vi "CC Hardware Config Dialog.vi"() -> (3 "Hardware Config":T1)   [LabVIEW 2024]
uses:
  typedefs/CC cluster Hardware Config.ctl
  typedefs/CC cluster Device Index.ctl
panel:
  in  "Edit":bool
  in  "Remove Type":bool
  in  "Add New Type":bool
  in  "Update":bool
  in  "Types":u16(ring) items=["Simulation", "RIMAS"]
  in  "Installed Hardware":i32(listbox)
  in  "Cancel Button":bool
  in  "OK Button":bool
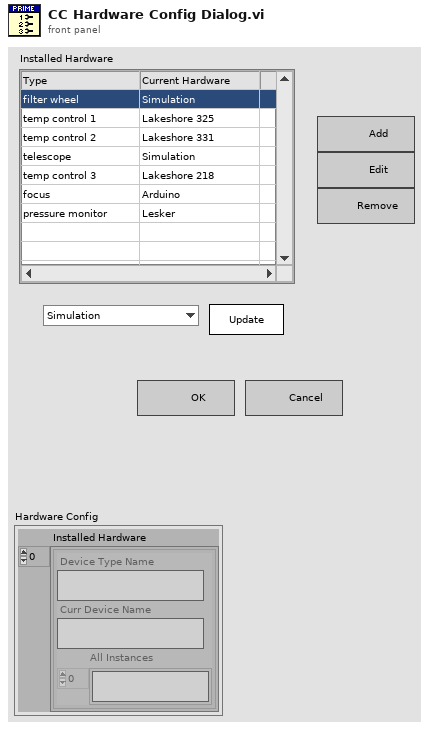
[diagram p1: front panel]
types:
  T1 = typedef "CC cluster Hardware Config.ctl" = cluster{"Installed Hardware":T2[]}
  T2 = typedef "CC cluster Device Index.ctl" = cluster{"Device Type Name":string, "Curr Device Name":string, "All Instances":string[]}
  T3 = cluster{"state":refnum<user-event>, "Hardware Config":T1}
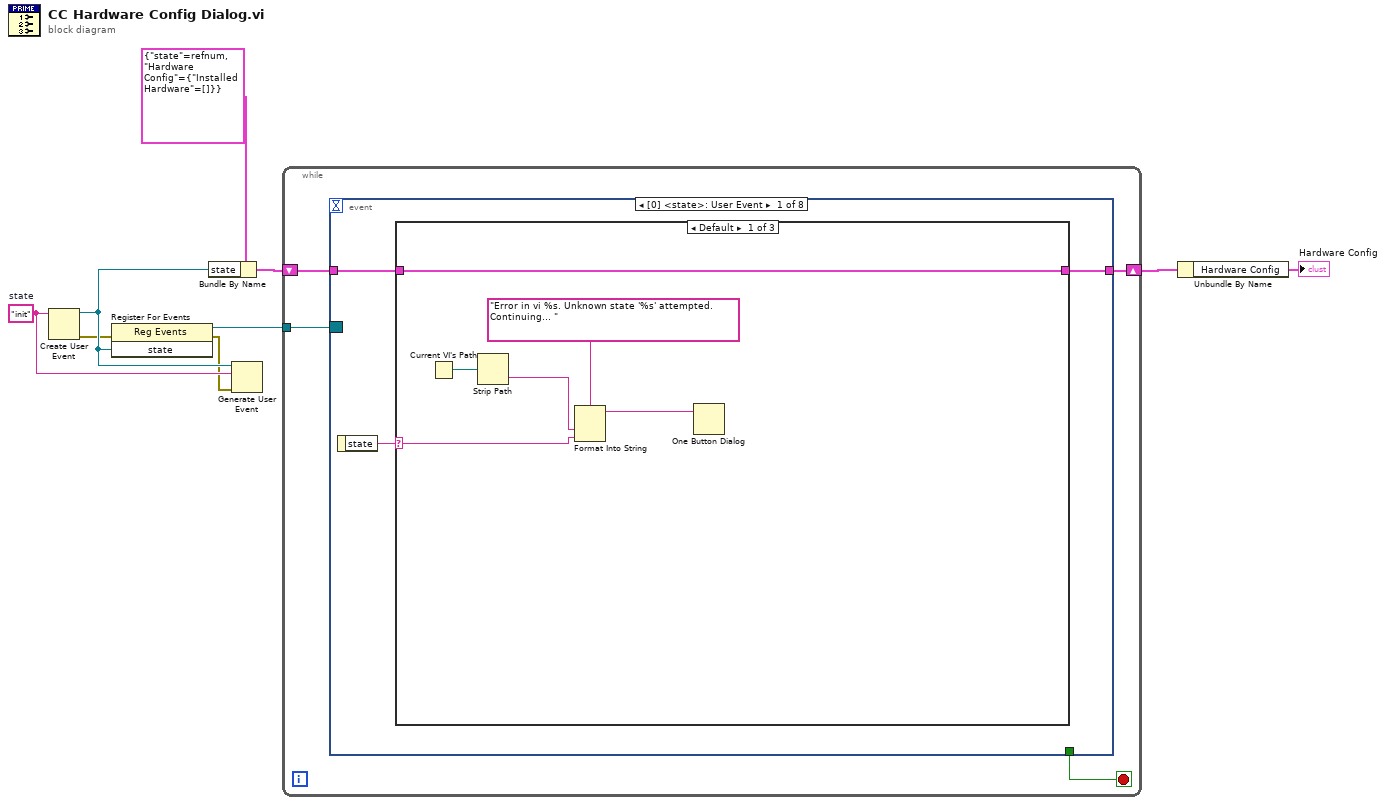
[diagram p0: block diagram]
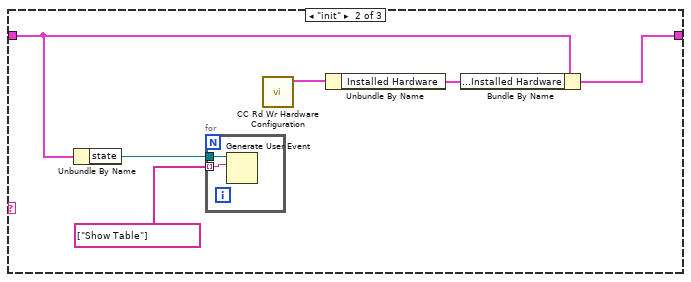
[diagram p2: hidden frame]
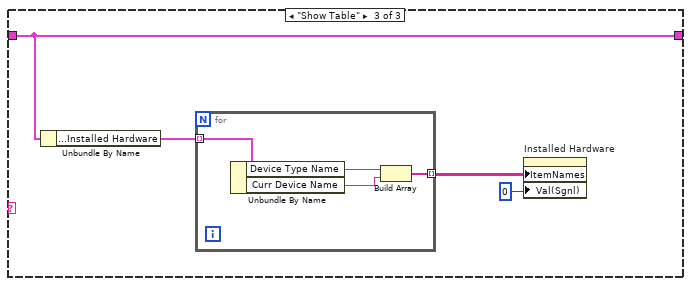
[diagram p3: hidden frame]
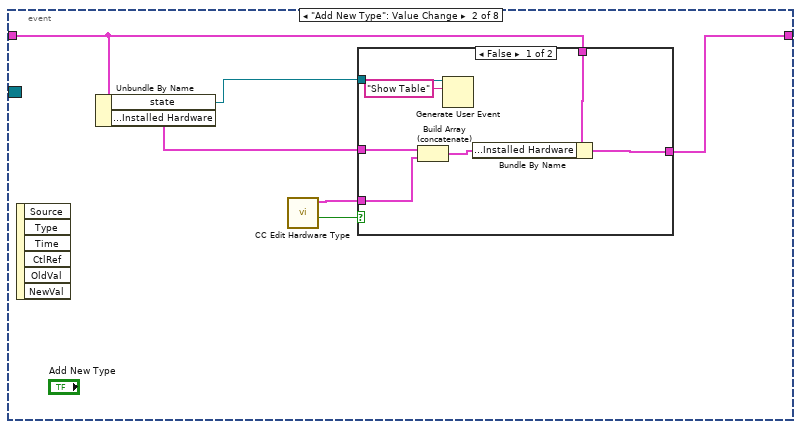
[diagram p4: hidden frame]
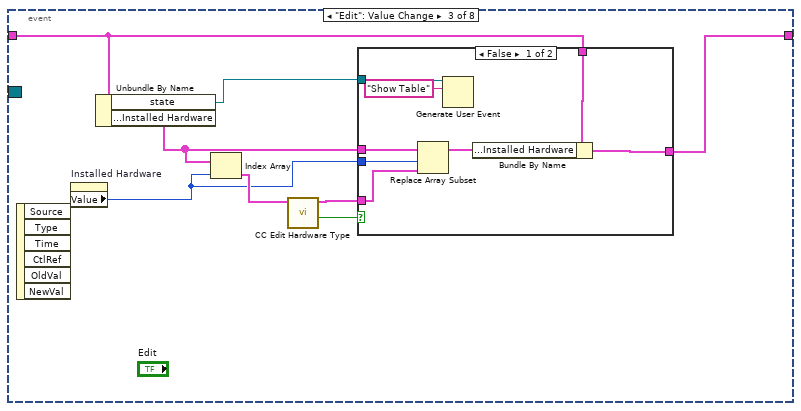
[diagram p6: hidden frame]
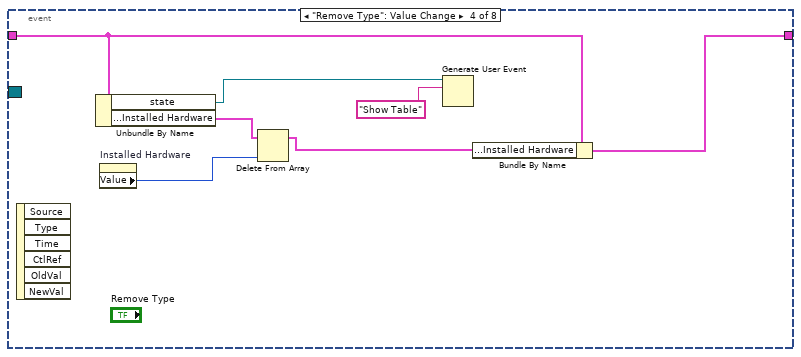
[diagram p8: hidden frame]
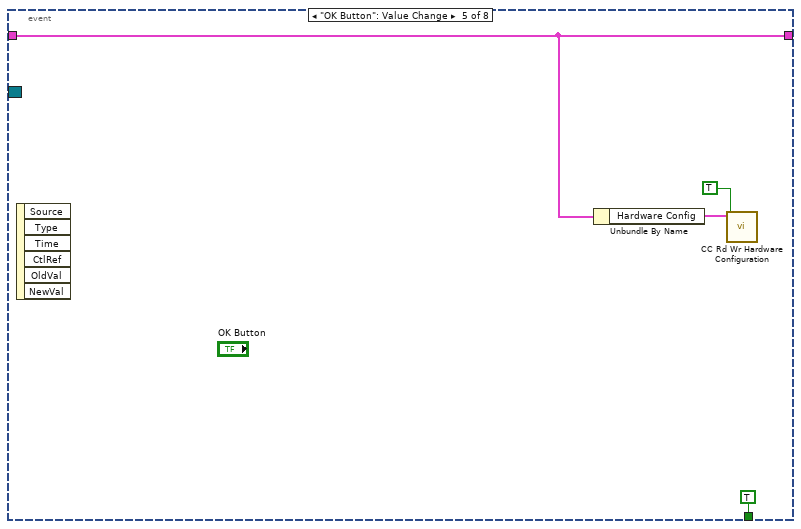
[diagram p9: hidden frame]
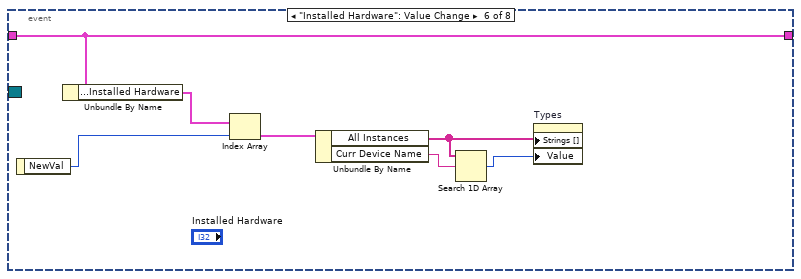
[diagram p10: hidden frame]
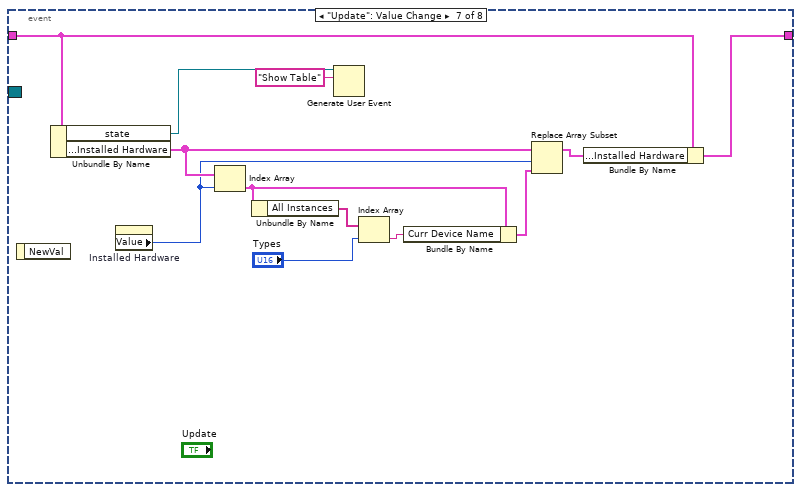
[diagram p11: hidden frame]
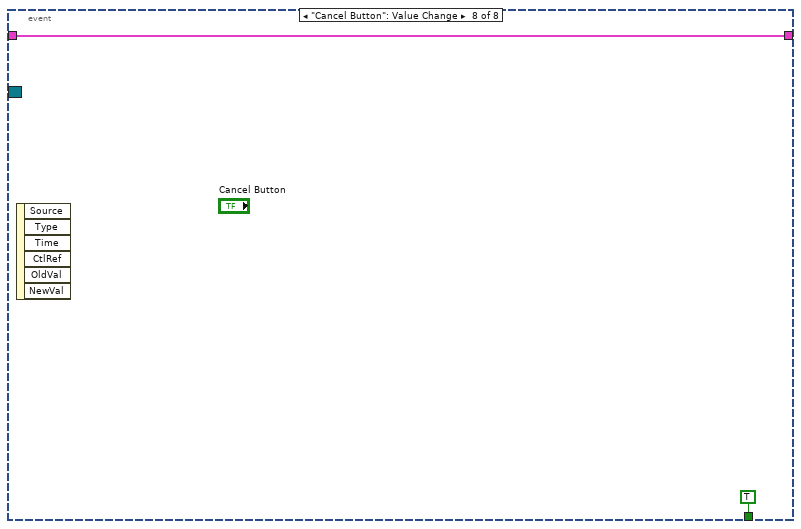
[diagram p12: hidden frame]
diagram:
  w5 = "init"  # state
  n1 = Create User Event(user event datatype=w5) -> (user event=w7:refnum<user-event>, error out=w3:errorcluster)  [unwired: 1 in]
  n2 = register-events(error in=w3, w7) -> (reference out=w6:refnum<event-registration>, error out=w4:errorcluster)  [unwired: 1 in]
  n3 = Bundle By Name(cluster=T3 {"state"=refnum, "Hardware Config"={"Installed Hardware"=[]}}, "state"=w7) -> (w8:T3)
  n4 = Generate User Event(user event=w7, event data cluster=w5, error in=w4) -> ()  [unwired: 1 in, 2 out]
  n5 = while {
    tunnel: w6 -> [w13]
    shift-right: [w11] -> w2
    shift-left: w8 -> [w12]
    stop <- w10 stop-if-true
    n6 = event shown="[0] <state>: User Event" {
      selector: w13 -> [_ _ _ _ _ _ _ _]
      dyn-events: _ -> [_ _ _ _ _ _ _ _]
      timeout: _ -> [_ _ _ _ _ _ _ _]
      tunnel: w12 -> [w15 w40 w57 w75 w77 w87 w90 w101]
      tunnel: [w14 w41 w58 w76 w77 w87 w91 w101] -> w11
      tunnel: [_ _ _ _ TRUE ("Close") _ _ TRUE ("Close")] -> w10
      event User Event {
        n7 = event-data() -> ("state"=w16:string)  [unwired: 1 in]
        n8 = case shown="Default" w16 {
          selector: w16 -> [w21 _ _]
          tunnel: w15 -> [w17 w25 w32]
          tunnel: [w17 w26 w32] -> w14
          frame Default {
            n9 = Current VI's Path() -> (path=w20:path)
            n10 = Strip Path(path=w20) -> (name=w19:string)  [unwired: 1 out]
            n11 = Format Into String(format string="Error in vi %s. Unknown state '%s' attempted. Continuing... ", w19, w21) -> (resulting string=w18:string)  [unwired: 2 in, 1 out]
            n12 = One Button Dialog(message=w18) -> ()  [unwired: 1 in, 1 out]
          }
          frame "init" {
            n13 = Unbundle By Name(w25) -> ("state"=w24:refnum<user-event>)
            n14 = for {
              tunnel: w24 -> [w30]
              tunnel: string[] ["Show Table"] -> [w29] mode=indexing
              n15 = Generate User Event(user event=w30, event data cluster=w29) -> ()  [unwired: 2 in, 2 out]
            }
            n16 = call "CC Rd Wr Hardware Configuration.vi"() -> ("Hardware Config out"=w28:T1)  [unwired: 8 in, 3 out]
            n17 = Unbundle By Name(w28) -> ("Installed Hardware"=w27:T2[])
            n18 = Bundle By Name(cluster=w25, "Hardware Config.Installed Hardware"=w27) -> (w26:T3)
          }
          frame "Show Table" {
            n19 = Unbundle By Name(w32) -> ("Hardware Config.Installed Hardware"=w34:T2[])
            n20 = for {
              tunnel: w34 -> [w38] mode=indexing
              tunnel: [w35] -> w33 mode=indexing
              n21 = Unbundle By Name(w38) -> ("Device Type Name"=w37:string, "Curr Device Name"=w36:string)
              n22 = Build Array(w37, w36) -> (w35:string[])
            }
            n23 = property on="Installed Hardware" class="MCListbox (strict)"("ItemNames"=w33, "Val(Sgnl)"=0 ("Value (Signaling)")) -> ()  [unwired: 2 in, 2 out]
          }
        }
      }
      event "Add New Type": Value Change {
        n24 = event-data() -> ()  [unwired: 1 in, 6 out]
        n25 = Unbundle By Name(w40) -> ("state"=w39:refnum<user-event>, "Hardware Config.Installed Hardware"=w42:T2[])
        n26 = call "CC Edit Hardware Type.vi"() -> ("cancelled?"=w44:bool, "Device out"=w43:T2)  [unwired: 9 in, 1 out]
        n27 = case shown="False" w44 {
          tunnel: w43 -> [w50 _]
          tunnel: w42 -> [w51 _]
          tunnel: w40 -> [w49 w52]
          tunnel: [w47 w52] -> w41
          tunnel: w39 -> [w46 _]
          frame False {
            n28 = Build Array (concatenate)(w51, w50) -> (w48:T2[])
            n29 = Generate User Event(user event=w46, event data cluster="Show Table" ("event data")) -> ()  [unwired: 2 in, 2 out]
            n30 = Bundle By Name(cluster=w49, "Hardware Config.Installed Hardware"=w48) -> (w47:T3)
          }
          frame True {
          }
        }
      }
      event "Edit": Value Change {
        n31 = event-data() -> ()  [unwired: 1 in, 6 out]
        n32 = property on="Installed Hardware" class="MCListbox (strict)"() -> ("Value"=w53:i32)  [unwired: 2 in, 2 out]
        n33 = Unbundle By Name(w57) -> ("state"=w56:refnum<user-event>, "Hardware Config.Installed Hardware"=w55:T2[])
        n34 = Index Array(array=w55, index=w53) -> (element=w54:T2)
        n35 = call "CC Edit Hardware Type.vi"("Device"=w54) -> ("cancelled?"=w60:bool, "Device out"=w59:T2)  [unwired: 8 in, 1 out]
        n36 = case shown="False" w60 {
          tunnel: w59 -> [w62 _]
          tunnel: w55 -> [w68 _]
          tunnel: w57 -> [w67 w69]
          tunnel: [w65 w69] -> w58
          tunnel: w56 -> [w64 _]
          tunnel: w53 -> [w61 _]
          frame False {
            n37 = Replace Array Subset(array=w68, new element=w62, index=w61) -> (w66:T2[])
            n38 = Generate User Event(user event=w64, event data cluster="Show Table" ("event data")) -> ()  [unwired: 2 in, 2 out]
            n39 = Bundle By Name(cluster=w67, "Hardware Config.Installed Hardware"=w66) -> (w65:T3)
          }
          frame True {
          }
        }
      }
      event "Remove Type": Value Change {
        n40 = event-data() -> ()  [unwired: 1 in, 6 out]
        n41 = Unbundle By Name(w75) -> ("state"=w74:refnum<user-event>, "Hardware Config.Installed Hardware"=w72:T2[])
        n42 = property on="Installed Hardware" class="MCListbox (strict)"() -> ("Value"=w73:i32)  [unwired: 2 in, 2 out]
        n43 = Delete From Array(array=w72, index=w73) -> (array with subset deleted=w70:T2[])  [unwired: 1 in, 1 out]
        n44 = Generate User Event(user event=w74, event data cluster="Show Table" ("event data")) -> ()  [unwired: 2 in, 2 out]
        n45 = Bundle By Name(cluster=w75, "Hardware Config.Installed Hardware"=w70) -> (w76:T3)
      }
      event "OK Button": Value Change {
        n46 = event-data() -> ()  [unwired: 1 in, 6 out]
        n47 = Unbundle By Name(w77) -> ("Hardware Config"=w80:T1)
        n48 = call "CC Rd Wr Hardware Configuration.vi"("Write? (F:Read)"=TRUE, "Hardware Config"=w80) -> ()  [unwired: 6 in, 4 out]
      }
      event "Installed Hardware": Value Change {
        n49 = event-data() -> ("NewVal"=w85:i32)  [unwired: 1 in]
        n50 = Unbundle By Name(w87) -> ("Hardware Config.Installed Hardware"=w86:T2[])
        n51 = Index Array(array=w86, index=w85) -> (element=w84:T2)
        n52 = Unbundle By Name(w84) -> ("All Instances"=w83:string[], "Curr Device Name"=w82:string)
        n53 = Search 1D Array(1D array=w83, element=w82) -> (index of element=w81:i32)  [unwired: 1 in]
        n54 = property on="Types" class="Ring (strict)"("Strings []"=w83, "Value"=w81) -> ()  [unwired: 2 in, 2 out]
      }
      event "Update": Value Change {
        n55 = event-data() -> ()  [unwired: 1 in, 1 out]
        n56 = Unbundle By Name(w90) -> ("state"=w89:refnum<user-event>, "Hardware Config.Installed Hardware"=w95:T2[])
        n57 = property on="Installed Hardware" class="MCListbox (strict)"() -> ("Value"=w94:i32)  [unwired: 2 in, 2 out]
        n58 = Index Array(array=w95, index=w94) -> (element=w97:T2)
        n59 = Unbundle By Name(w97) -> ("All Instances"=w99:string[])
        n60 = Generate User Event(user event=w89, event data cluster="Show Table" ("event data")) -> ()  [unwired: 2 in, 2 out]
        n61 = Index Array(array=w99, index="Types") -> (element=w96:string)
        n62 = Bundle By Name(cluster=w97, "Curr Device Name"=w96) -> (w93:T2)
        n63 = Replace Array Subset(array=w95, new element=w93, index=w94) -> (w92:T2[])
        n64 = Bundle By Name(cluster=w90, "Hardware Config.Installed Hardware"=w92) -> (w91:T3)
      }
      event "Cancel Button": Value Change {
        n65 = event-data() -> ()  [unwired: 1 in, 6 out]
      }
    }
  }
  n66 = Unbundle By Name(w2) -> ("Hardware Config"=→"Hardware Config":T1)
